vi "Prorject4.vi"() -> ()   [LabVIEW 2024]
panel:
  in  "COMM_Name":refnum<visa-resource-name>
  in  "stop":bool
  out "Warm":bool
  out "Cold":bool
  out "Waveform Chart":dbl(graph)
  out "Thermometer, C":dbl(slide) scale=0.0..100.0
  out "R, KOhms":dbl format="%1.2f"
  out "AtoD, Hex":i32 format="%04x"
  out "SCC, V":dbl format="%01.3f"
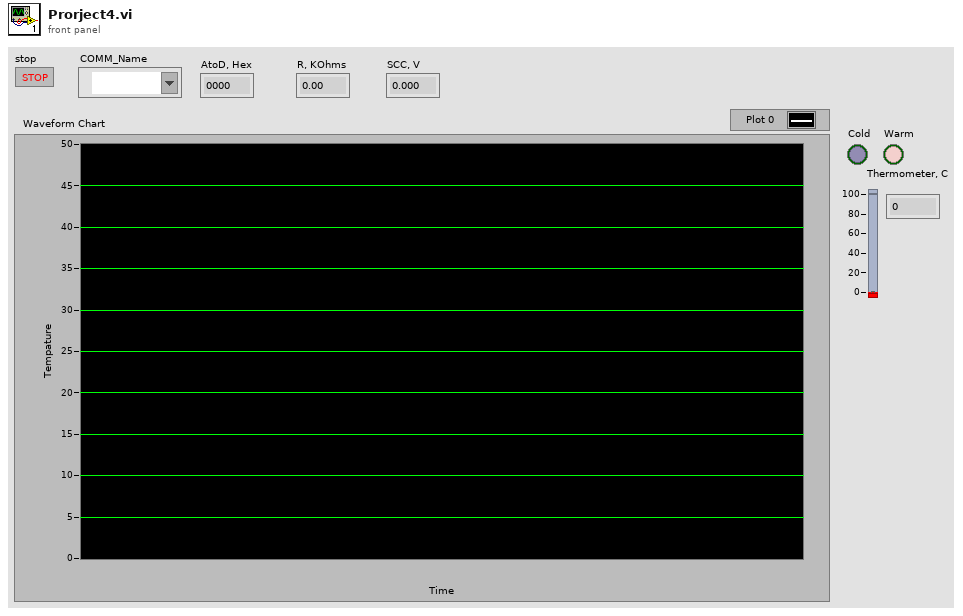
[diagram p1: front panel]
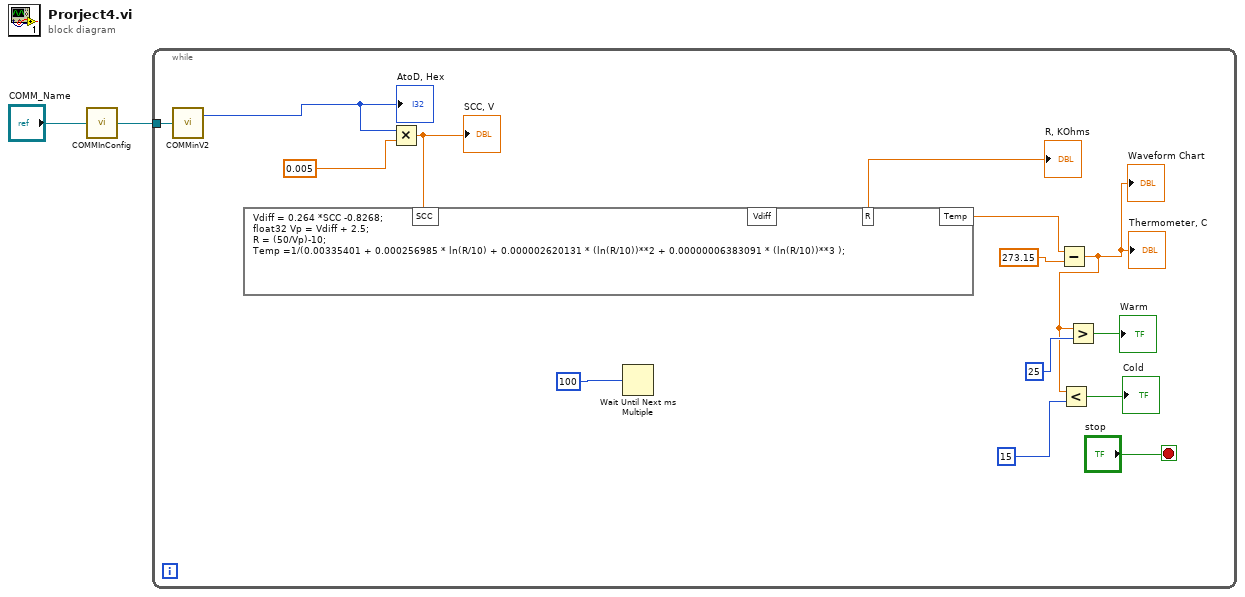
[diagram p0: block diagram]
diagram:
  n1 = call "COMMInConfig.vi"("COMM_in"="COMM_Name") -> ("COMM_Name"=w2:refnum<visa-resource-name>)
  n2 = while {
    tunnel: w2 -> [w6]
    stop <- "stop" stop-if-true
    n3 = call "COMMinV2.vi"("VISA resource name"=w6) -> ("AtoDOut"=w5:i16)  [unwired: 1 out]
    "AtoD, Hex" <- w5
    n4 = Multiply(x=w5, y=0.005) -> (x*y=w16:dbl)
    "SCC, V" <- w16
    n5 = formula code="Vdiff = 0.264 *SCC -0.8268;\nfloat32 Vp = Vdiff + 2.5;\nR = (50/Vp)-10;\nTemp =1/(0.00335401 + 0.000256985 * ln(R/10) + 0.000002620131 * (ln(R/10))**2 + 0.00000006383091 * (ln(R/10))**3 );"("SCC"=w16) -> ("R"=→"R, KOhms":dbl, "Temp"=w4:dbl)  [unwired: 1 out]
    n6 = Wait Until Next ms Multiple(millisecond multiple=100) -> ()  [unwired: 1 out]
    n7 = Subtract(x=w4, y=273.15) -> (x-y=w3:dbl)
    "Thermometer, C" <- w3
    "Waveform Chart" <- w3
    n8 = Less?(x=w3, y=15) -> (x < y?=→"Cold":bool)
    n9 = Greater?(x=w3, y=25) -> (0:→"Warm":bool)
  }
